vi "Measurement Parameters.vi"(8 "error in (no error)":errorcluster, 10 "Number Of Meas Points (400)":i32=400, 11 "VISA resource name":refnum<visa-resource-name>) -> (0 "error out":errorcluster, 3 "VISA resource name out":refnum<visa-resource-name>)   [LabVIEW 2010, in "Agilent 4194.lvlib"]
doc: "This function specifies the measure parameter - number of measured points."
uses:
  <instrlib>/Agilent 4194/Agilent 4194.lvlib
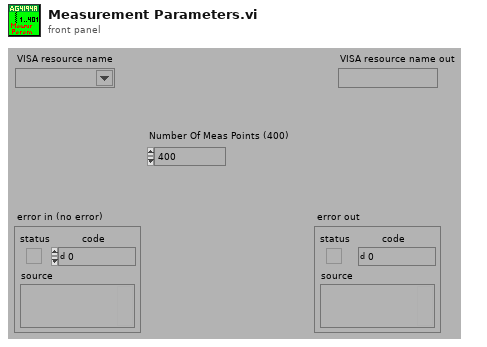
[diagram p1: front panel]
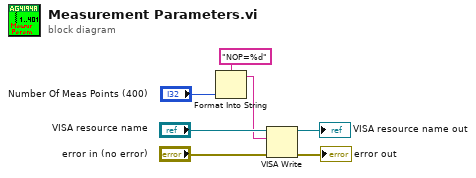
[diagram p0: block diagram]
diagram:
  n1 = Format Into String(format string="NOP=%d", "Number Of Meas Points (400)") -> (resulting string=w1:string)  [unwired: 2 in, 1 out]
  n2 = VISA Write(VISA resource name="VISA resource name", write buffer=w1, error in (no error)="error in (no error)") -> (VISA resource name out=→"VISA resource name out":refnum<visa-resource-name>, error out=→"error out":errorcluster)  [unwired: 1 out]
